vi "Create Channel.vi"(7 "Ranges":T2[](array[typedef]), 8 "error in (no error)":errorcluster, 9 "Buffer size":i32=1000, 10 "Phisical channels":T1[](array[typedef]) items=["AO1"=1, "AO2"=2, "AO3"=3, "AO4"=4, "AO5"=5, "AO6"=6, "AO7"=7, "AO8"=8, "AO9"=9, "AO10"=10, "AO11"=11, "AO12"=12, "AO13"=13, "AO14"=14, "AO15"=15, "AO16"=16], 11 "Connection ID":i32=-1) -> (0 "error out":errorcluster, 3 "Task Out":refnum<class "Analog output.lvclass">)   [LabVIEW 2009, in "MicroDAQ.lvlib" / "Analog output.lvclass"]
doc: "Creates channel(s) to generate voltage. Queued data size must be the equal to specfied Buffor size.\n\nUse Configure channel.VI to specify Sample Rate, Mode and other settings."
uses:
  <instrlib>/MicroDAQ/Channel/Analog Output/Analog output.lvclass
  <instrlib>/MicroDAQ/Tools/Analo Range Enum.ctl
  <instrlib>/MicroDAQ/Tools/Analog Channel Enum.ctl
  <instrlib>/MicroDAQ/Channel/Analog Output/Analog output.lvclass/Analog output.ctl
  <instrlib>/MicroDAQ/Channel/Channel.lvclass
  <instrlib>/MicroDAQ/MicroDAQ.lvlib
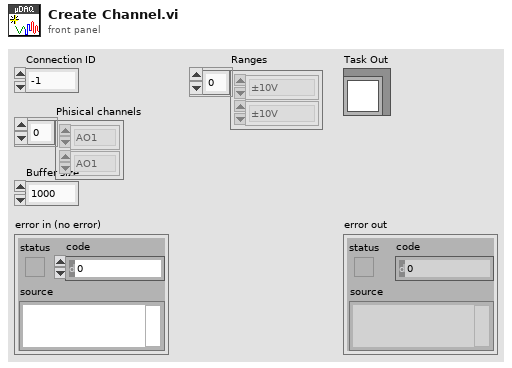
[diagram p1: front panel]
types:
  T1 = typedef "MicroDAQ.lvlib/Analog Channel Enum.ctl" = u16
  T2 = typedef "MicroDAQ.lvlib/Analo Range Enum.ctl" = enum16{"±10V", "0-10V", "±5V", "0-5V", "±5.12V", "±2.56V", "±2.5V", "±2V", "±1.24V", "±0.64V"}
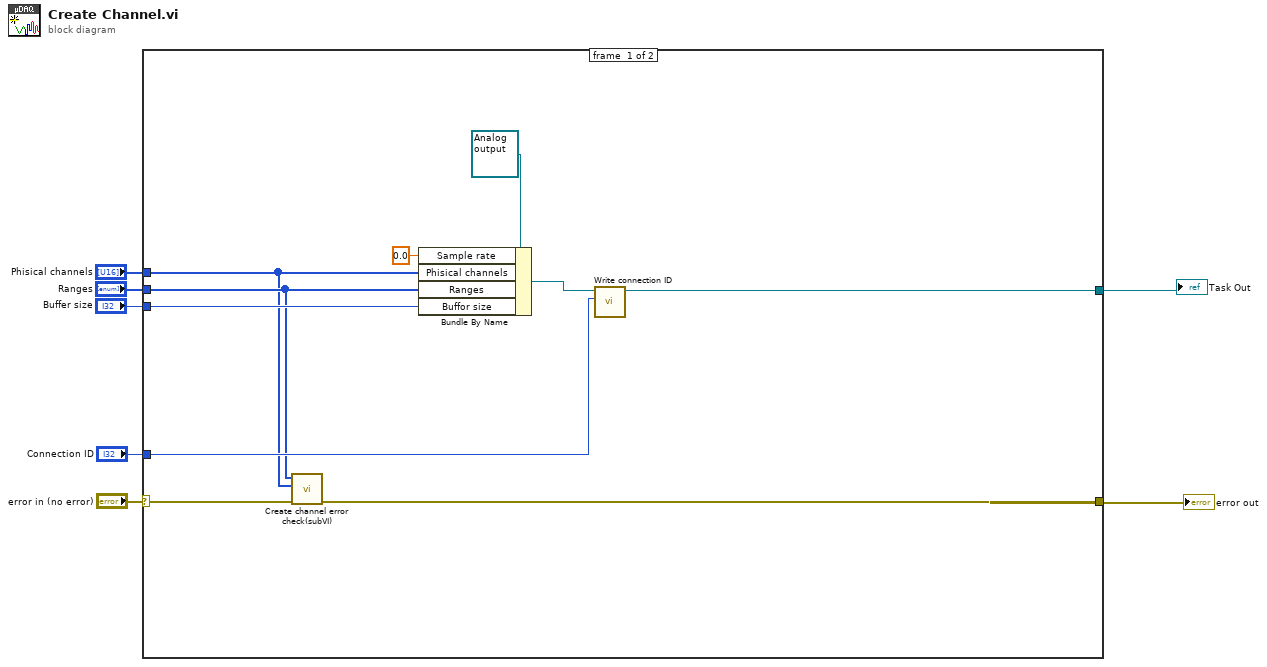
[diagram p0: block diagram]
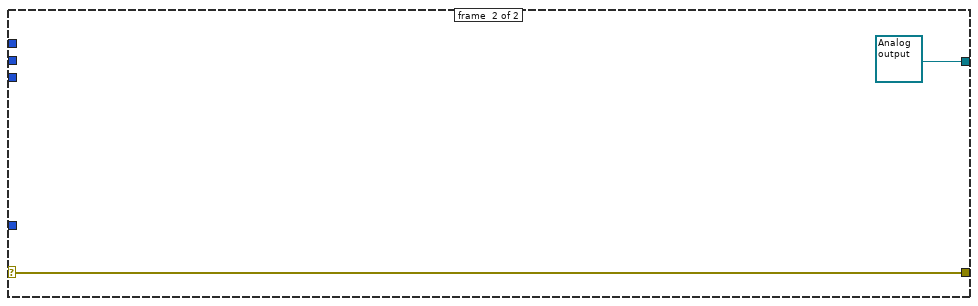
[diagram p2: hidden frame]
diagram:
  n1 = case shown="No Error" "error in (no error)" {
    selector: "error in (no error)" -> [w12 w19]
    tunnel: [w9 w19] -> w6
    tunnel: "Phisical channels" -> [w10 _]
    tunnel: "Ranges" -> [w11 _]
    tunnel: "Buffer size" -> [w16 _]
    tunnel: "Connection ID" -> [w13 _]
    tunnel: [w14 refnum<class "Analog output.lvclass"> refnum ("MicroDAQ.lvlib:Analog Output.lvclass")] -> w1
    frame #0 {
      n2 = call <instrlib>:"Create channel error check(subVI).vi"("error in (no error)"=w12, "Phisical channels"=w10, "Ranges"=w11) -> ("error out"=w9:errorcluster)  [unwired: 8 in]
      n3 = Bundle By Name(cluster=refnum<class "Analog output.lvclass"> refnum ("MicroDAQ.lvlib:Analog Output.lvclass"), "Sample rate"=0.0, "Phisical channels"=w10, "Ranges"=w11, "Buffor size"=w16) -> (w15:refnum<class "Analog output.lvclass">)
      n4 = call <instrlib>:"Write connection ID.vi"("connection ID"=w13, "Task in"=w15) -> ("Task out"=w14:refnum<class "Analog output.lvclass">)  [unwired: 9 in]
    }
    frame #1 {
    }
  }
  "Task Out" <- w1
  "error out" <- w6
